vi "Get Timing Section Reference.vi"(8 "error in":errorcluster, 11 "Custom device Ref":T1 format="%.0x") -> (0 "error out":errorcluster, 1 "Found":bool, 3 "Custom device Ref out":T1 format="%.0x")   [LabVIEW 2020, in "Communication Bus Template Scripting.lvlib"]
uses:
  <vilib>/NI VeriStand/Custom Device API/Custom Device Item Ref.ctl
  Constants.vi
  Communication Bus Template Scripting.lvlib
  <vilib>/NI VeriStand/Custom Device Tools/Custom Device Utility Library/Custom Device Utility Library.lvlib
  <vilib>/NI VeriStand/Custom Device Tools/Custom Device Utility Library/NI VeriStand - Search for Item by GUID.vi
  <vilib>/NI VeriStand/Custom Device API/Custom Device API.lvlib
panel:
  out "Timing section Ref":T1=18446744073709551615 format="%.0x"
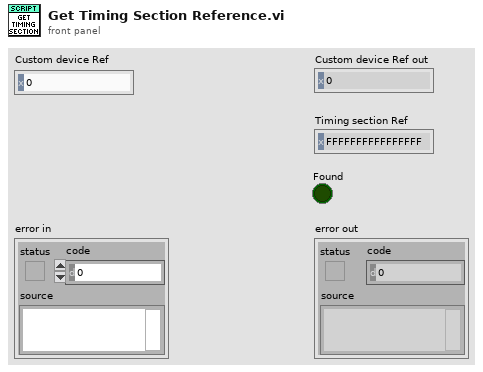
[diagram p1: front panel]
types:
  T1 = typedef "Custom Device API.lvlib/Custom Device Item Ref.ctl" = u64
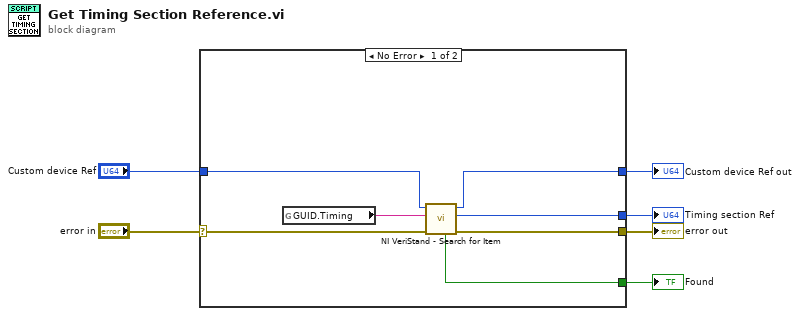
[diagram p0: block diagram]
diagram:
  n1 = case shown="No Error" "error in" {
    selector: "error in" -> [w12 w15]
    tunnel: "Custom device Ref" -> [w11 w14]
    tunnel: [w8 w15] -> w5
    tunnel: [w10 w14] -> w3
    tunnel: [w9 _] -> w2
    tunnel: [w7 _] -> w1
    frame No Error {
      n2 = global read "Constants.vi" "GUID.Timing"() -> (w13:string)
      n3 = call-poly <vilib>:"NI VeriStand - Search for Item.vi"("error in"=w12, "Item GUID"=w13, "Section Ref in"=w11) -> ("error out"=w8:errorcluster, "Item Ref"=w9:T1, "Section Ref out"=w10:T1, "Found"=w7:bool)  [unwired: 5 in]
    }
    frame Error {
    }
  }
  "error out" <- w5
  "Custom device Ref out" <- w3
  "Timing section Ref" <- w2
  "Found" <- w1
